vi "KupaSurahiKontrol.vi"(7 "Çarpan":dbl, 8 "Kahve":dbl, 9 "Çay":dbl, 10 "Su":dbl, 11 "içicek":i64) -> (0 "Kahve çýkýþ":dbl, 1 "Çay çýkýþ":dbl, 2 "Su çýkýþ":dbl)   [LabVIEW 2021]
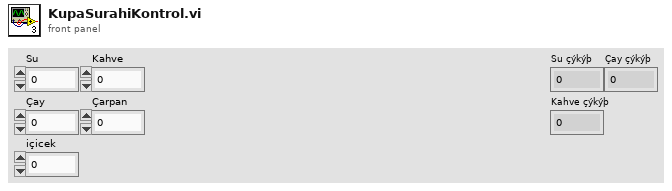
[diagram p1: front panel]
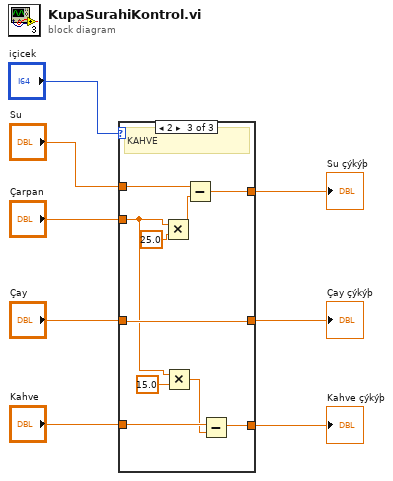
[diagram p0: block diagram]
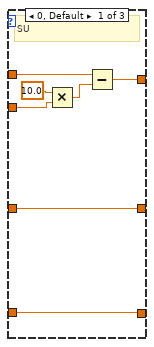
[diagram p2: hidden frame]
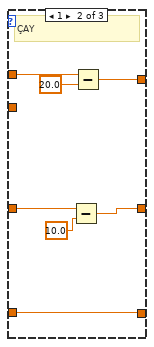
[diagram p3: hidden frame]
diagram:
  n1 = case shown="2" "içicek" {
    tunnel: "Su" -> [w15 w22 w32]
    tunnel: "Çay" -> [w13 w20 w30]
    tunnel: "Kahve" -> [w12 w16 w31]
    tunnel: [w14 w18 w29] -> w4
    tunnel: [w13 w17 w30] -> w3
    tunnel: [w12 w16 w28] -> w2
    tunnel: "Çarpan" -> [w9 _ w23]
    frame 0, Default {
      # "SU"
      n2 = Multiply(x=10.0 ("y"), y=w9) -> (x*y=w10:dbl)
      n3 = Subtract(x=w15, y=w10) -> (x-y=w14:dbl)
    }
    frame 1 {
      # "ÇAY"
      n4 = Subtract(x=w20, y=10.0) -> (x-y=w17:dbl)
      n5 = Subtract(x=w22, y=20.0) -> (x-y=w18:dbl)
    }
    frame 2 {
      # "KAHVE"
      n6 = Multiply(x=w23, y=25.0) -> (x*y=w26:dbl)
      n7 = Multiply(x=w23, y=15.0) -> (x*y=w24:dbl)
      n8 = Subtract(x=w32, y=w26) -> (x-y=w29:dbl)
      n9 = Subtract(x=w31, y=w24) -> (x-y=w28:dbl)
    }
  }
  "Su çýkýþ" <- w4
  "Çay çýkýþ" <- w3
  "Kahve çýkýþ" <- w2
